vi "Get_Type.vi"(8 "error in (no error)":errorcluster, 11 ".NET Reference in":refnum<k24>) -> (0 "error out":errorcluster, 2 "type":string, 3 "Reference out":refnum<k24>)   [LabVIEW 2017]
uses:
  D:/test/FULLband-sts/Fullband_Sample/DLL/InstrumentDLL.dll
  DLL/InstrumentDLL.dll
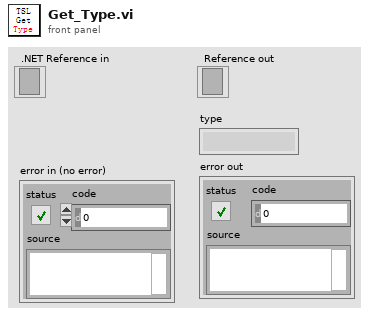
[diagram p1: front panel]
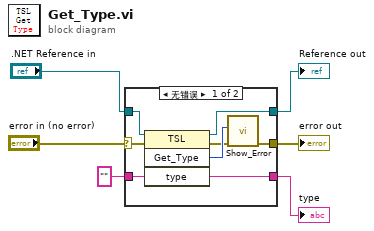
[diagram p0: block diagram]
diagram:
  n1 = case shown="无错误" "error in (no error)" {
    selector: "error in (no error)" -> [w7 w16]
    tunnel: ".NET Reference in" -> [w14 w17]
    tunnel: [w13 w17] -> w5
    tunnel: [w8 w16] -> w4
    tunnel: "" ("type") -> [w12 w15]
    tunnel: [w11 w15] -> w2
    frame No Error {
      n2 = invoke on="调用节点" class="TSL" method="Get_Type"(reference=w14, error in=w7, "type"=w12) -> (reference out=w13:refnum<k24>, error out=w9:errorcluster, "Get_Type"=w10:i32, "type"=w11:string)  [unwired: 1 in]
      n3 = call "Show_Error.vi"("error in (no error)"=w9, "Error"=w10) -> ("error out"=w8:errorcluster)  [unwired: 9 in]
    }
    frame Error {
    }
  }
  "Reference out" <- w5
  "error out" <- w4
  "type" <- w2
